vi "SecondaryData.vi"(9 "Variant":variant, 10 "Input":dbl[](array[numeric]), 11 "Option":i32) -> (2 "SecondaryData":dbl[](array[numeric]))   [LabVIEW 2014, in "GenericDAQ.lvlib"]
uses:
  <instrlib>/GenericDAQ/GenericDAQ.lvlib
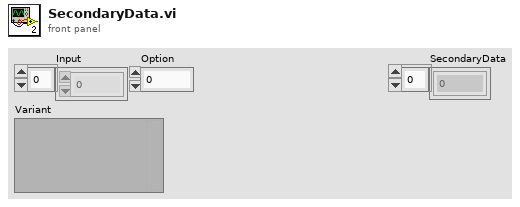
[diagram p1: front panel]
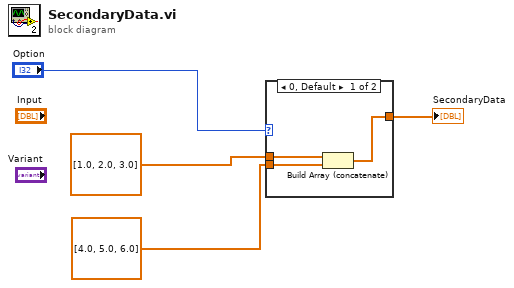
[diagram p0: block diagram]
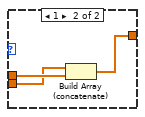
[diagram p2: hidden frame]
diagram:
  n1 = case shown="0, Default" "Option" {
    tunnel: dbl[] [1.0, 2.0, 3.0] ("Position(Micos)") -> [w7 w10]
    tunnel: dbl[] [4.0, 5.0, 6.0] ("Position_ESP") -> [w6 w9]
    tunnel: [w5 w8] -> w4
    frame 0, Default {
      n2 = Build Array (concatenate)(w7, w6) -> (w5:dbl[])
    }
    frame 1 {
      n3 = Build Array (concatenate)(w9, w10) -> (w8:dbl[])
    }
  }
  "SecondaryData" <- w4
